vi "Capture@AddCAM__Parameter.vi"(1 "ParamterIn":string) -> (0 "ParamterOut":string)   [LabVIEW 2020]
uses:
  MainFrame/Global.vi
panel:
  out "Example Setting":string
  in  "Others":string(combo)
  in  "Driver":string(combo)="NIVAS"
  in  "CamName":string(combo)
  in  "Confirm":bool
  # "Capture@AddCAM $Capture,$Driver(,Parameter)"
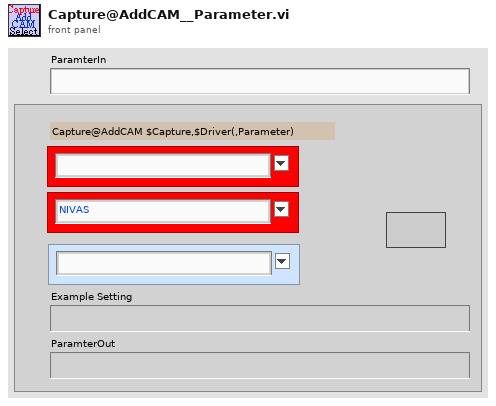
[diagram p1: front panel]
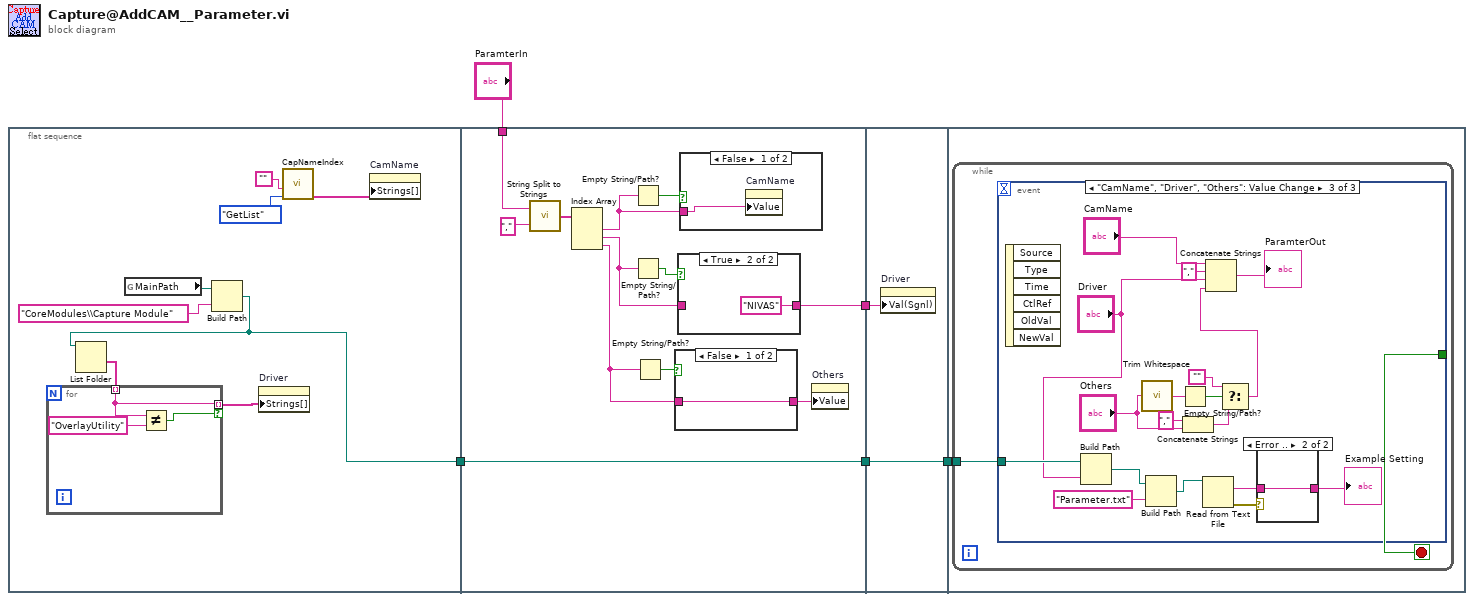
[diagram p0: block diagram]
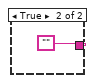
[diagram p2: hidden frame]
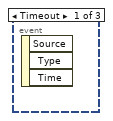
[diagram p5: hidden frame]
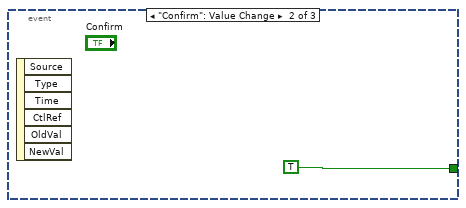
[diagram p6: hidden frame]
diagram:
  n1 = flat-sequence {
    tunnel: [w6] -> w1
    tunnel: "ParamterIn" -> [w26]
    tunnel: [w18] -> w4
    tunnel: [w17] -> w2
    tunnel: w1 -> [w17]
    tunnel: w4 -> [w35]
    tunnel: [w34] -> w3
    tunnel: w2 -> [w34]
    tunnel: w3 -> [w36]
    frame #0 {
      n2 = global read "Global.vi" "MainPath"() -> (w10:path)
      n3 = Build Path(base path=w10, name or relative path="CoreModules\\Capture Module") -> (appended path=w6:path)
      n4 = List Folder(path=w6) -> (folder names=w8:string[])  [unwired: 3 in, 3 out]
      n5 = for {
        tunnel: w8 -> [w15] mode=indexing
        tunnel: [w15] -> w7 mode=indexing if=w14
        n6 = Not Equal?(x=w15, y="OverlayUtility") -> (x != y?=w14:bool)
      }
      n7 = property on="Driver" class="CmbBox"("Strings[]"=w7) -> ()  [unwired: 2 in, 2 out]
      n8 = call "CapNameIndex.vi"("OP"=enum16{"AddCam", "GetIndex", "Init", "GetList"}."GetList", "CamName"="") -> ("DeviceList"=w12:string[])  [unwired: 2 in, 3 out]
      n9 = property on="CamName" class="CmbBox"("Strings[]"=w12) -> ()  [unwired: 2 in, 2 out]
    }
    frame #1 {
      n10 = call "String Split to Strings.vi"("search string/char (-)"=",", "String"=w26) -> ("Array"=w28:string[])
      n11 = Index Array(array=w28) -> (element #1=w24:string, element #2=w22:string, element #3=w20:string)  [unwired: 3 in]
      n12 = Empty String/Path?(string/path=w24) -> (empty?=w25:bool)
      n13 = Empty String/Path?(string/path=w22) -> (empty?=w23:bool)
      n14 = Empty String/Path?(string/path=w20) -> (empty?=w21:bool)
      n15 = case shown="False" w21 {
        tunnel: [w29 ""] -> w19
        tunnel: w20 -> [w29 _]
        frame False {
        }
        frame True {
        }
      }
      n16 = case shown="True" w23 {
        tunnel: [w31 "NIVAS"] -> w18
        tunnel: w22 -> [w31 _]
        frame False {
        }
        frame True {
        }
      }
      n17 = case shown="False" w25 {
        tunnel: w24 -> [w33 _]
        frame False {
          n18 = property on="CamName" class="CmbBox"("Value"=w33) -> ()  [unwired: 2 in, 2 out]
        }
        frame True {
        }
      }
      n19 = property on="Others" class="CmbBox"("Value"=w19) -> ()  [unwired: 2 in, 2 out]
    }
    frame #2 {
      n20 = property on="Driver" class="CmbBox"("Val(Sgnl)"=w35) -> ()  [unwired: 2 in, 2 out]
    }
    frame #3 {
      n21 = while {
        tunnel: w36 -> [w37]
        stop <- w38 stop-if-true
        n22 = event shown="[2] \"CamName\", \"Driver\", \"Others\": Value Change" {
          selector: _ -> [_ _ _]
          dyn-events: _ -> [_ _ _]
          timeout: _ -> [_ _ _]
          tunnel: [_ TRUE _] -> w38
          tunnel: w37 -> [_ _ w47]
          event Timeout {
            n23 = event-data() -> ()  [unwired: 1 in, 3 out]
          }
          event "Confirm": Value Change {
            n24 = event-data() -> ()  [unwired: 1 in, 6 out]
          }
          event "CamName", "Driver", "Others": Value Change {
            n25 = event-data() -> ()  [unwired: 1 in, 6 out]
            n26 = Build Path(base path=w47, name or relative path="Driver") -> (appended path=w45:path)
            n27 = call <vilib>:"Trim Whitespace.vi"("string"="Others") -> ("trimmed string"=w51:string)  [unwired: 1 in]
            n28 = Build Path(base path=w45, name or relative path="Parameter.txt") -> (appended path=w43:path)
            n29 = Empty String/Path?(string/path=w51) -> (empty?=w52:bool)
            n30 = Concatenate Strings("," ("string"), "Others") -> (w54:string)
            n31 = Read from Text File(file (use dialog)=w43) -> (text=w41:string, error out=w42:errorcluster)  [unwired: 3 in, 2 out]
            n32 = Select(t="", s=w52, f=w54) -> (s? t:f=w49:string)
            n33 = Concatenate Strings("CamName", "," ("string"), "Driver", w49) -> (→"ParamterOut":string)
            n34 = case shown="Error .." w42 {
              tunnel: w41 -> [w58 w59]
              tunnel: [w58 w59] -> w40
              frame No Error {
              }
              frame Error {
              }
            }
            "Example Setting" <- w40
          }
        }
      }
    }
  }
